vi "make_path.vi"(11 "file_name":string) -> (3 "file path":path)   [LabVIEW 2009]
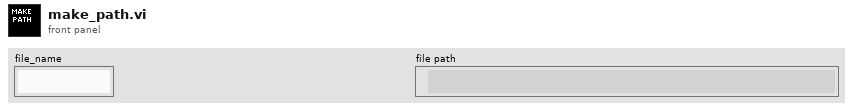
[diagram p1: front panel]
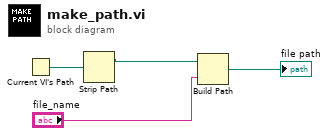
[diagram p0: block diagram]
diagram:
  n1 = Current VI's Path() -> (path=w2:path)
  n2 = Strip Path(path=w2) -> (stripped path=w1:path)  [unwired: 1 out]
  n3 = Build Path(base path=w1, name or relative path="file_name") -> (appended path=→"file path":path)
